vi "Record Recent User.vi"(8 "error in (no error)":errorcluster, 11 "[Data] Recent User in":refnum<class "[Data] Recent User.lvclass">) -> (0 "error out":errorcluster, 3 "[Data] Recent User out":refnum<class "[Data] Recent User.lvclass">)   [LabVIEW 2020, in "[Data] Recent User.lvclass"]
uses:
  [Data] Recent User.lvclass
  [Data] Recent User.lvclass/[Data] Recent User.ctl
  62142596-0b0f-4c2f-9c94-56f427fad02b.vi
  <vilib>/Comparison/Equal/Equal Functor/Equal Functor.lvclass
panel:
  in  "username":string
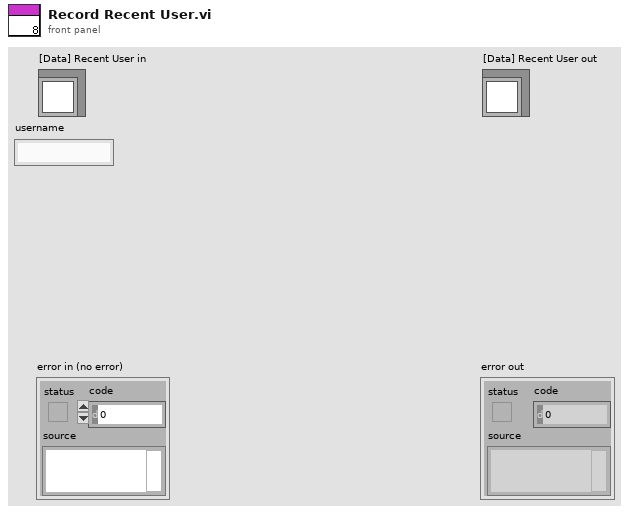
[diagram p1: front panel]
types:
  T1 = cluster{"enable rmb user":bool, "recent user list":string[]}
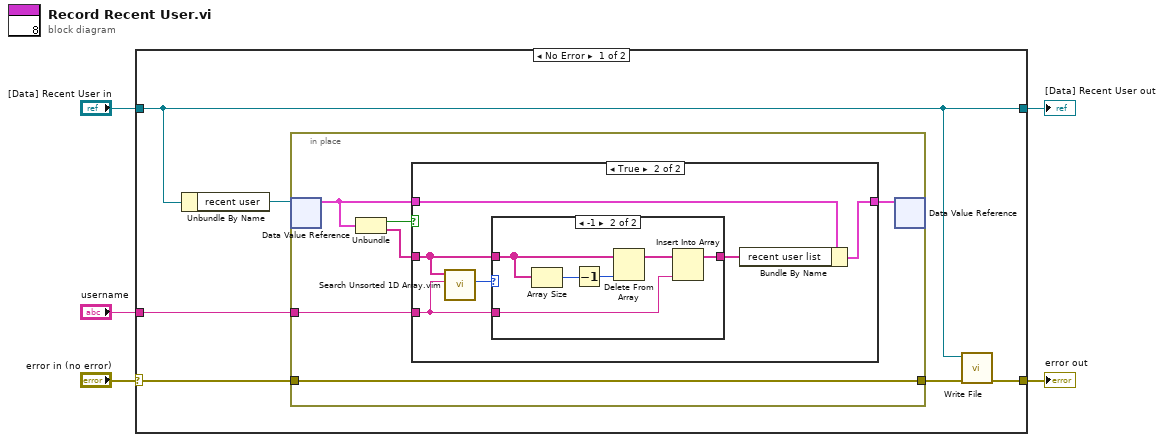
[diagram p0: block diagram]
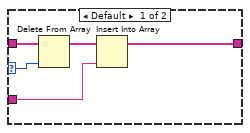
[diagram p3: hidden frame]
diagram:
  n1 = case shown="No Error" "error in (no error)" {
    selector: "error in (no error)" -> [w9 w37]
    tunnel: [w7 w37] -> w4
    tunnel: [w6 w36] -> w2
    tunnel: "[Data] Recent User in" -> [w6 w36]
    tunnel: "username" -> [w10 _]
    frame No Error {
      n2 = Unbundle By Name(w6) -> ("recent user"=w11:refnum<data-value>)
      n3 = in-place {
        in-place-border: w10 -> [w14]
        in-place-border: w9 -> [w12]
        in-place-border: [w12] -> w8
        n4 = in-place-dvr #1(w11) -> (w17:T1)  [unwired: 1 out]
        n5 = Unbundle(w17) -> ("enable rmb user"=w16:bool, "recent user list"=w15:string[])
        n6 = case shown="True" w16 {
          tunnel: w15 -> [_ w23]
          tunnel: w14 -> [_ w22]
          tunnel: w17 -> [w18 w21]
          tunnel: [w18 w19] -> w13
          frame False {
          }
          frame True {
            n7 = call "Search Unsorted 1D Array.vim"("element"=w22, "unsorted 1D array"=w23) -> ("index of element"=w24:i32)  [unwired: 9 in]
            n8 = case shown="-1" w24 {
              selector: w24 -> [w28 _]
              tunnel: w23 -> [w29 w35]
              tunnel: w22 -> [w26 w31]
              tunnel: [w25 w30] -> w20
              frame Default {
                n9 = Delete From Array(array=w29, index=w28) -> (array with subset deleted=w27:string[])  [unwired: 1 in, 1 out]
                n10 = Insert Into Array(array=w27, new element=w26) -> (w25:string[])  [unwired: 1 in]
              }
              frame -1 {
                n11 = Array Size(array=w35) -> (size(s)=w34:i32)
                n12 = Decrement(x=w34) -> (x-1=w33:i32)
                n13 = Delete From Array(array=w35, index=w33) -> (array with subset deleted=w32:string[])  [unwired: 1 in, 1 out]
                n14 = Insert Into Array(array=w32, new element=w31) -> (w30:string[])  [unwired: 1 in]
              }
            }
            n15 = Bundle By Name(cluster=w21, "recent user list"=w20) -> (w19:T1)
          }
        }
        n16 = in-place-dvr #1(w13) -> ()  [unwired: 2 out]
      }
      n17 = call "Write File.vi"("error in (no error)"=w8, "[Data] Recent User in"=w6) -> ("error out"=w7:errorcluster)  [unwired: 8 in, 1 out]
    }
    frame Error {
    }
  }
  "error out" <- w4
  "[Data] Recent User out" <- w2
